vi "visible.vi"(11 "station array":refnum<vi>[](array[refnum])) -> ()   [LabVIEW 2017]
panel:
  in  "reference":refnum<vi>
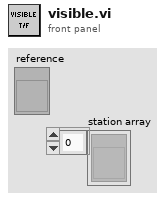
[diagram p1: front panel]
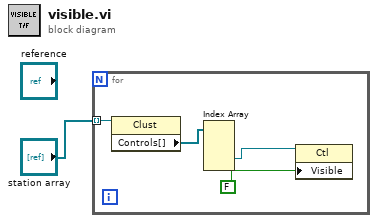
[diagram p0: block diagram]
diagram:
  n1 = for {
    tunnel: "station array" -> [w2] mode=indexing
    n2 = property on="Property Node" class="Clust"(reference=w2) -> ("Controls[]"=w3:refnum<vi>[])  [unwired: 1 in, 2 out]
    n3 = Index Array(array=w3) -> (element #3=w4:refnum<vi>)  [unwired: 4 in, 3 out]
    n4 = property class="Ctl"(reference=w4, "Visible"=FALSE) -> ()  [unwired: 1 in, 2 out]
  }
